vi "message_handle.vi"(0 "Host_Reference":refnum<class "HGF_Reference.lvclass">, 2 "MoAgSy_Message":refnum<class "MoAgSy_Message.lvclass">, 5 "error in (no error)":errorcluster, 8 "timeout in ms (-1)":i32=100) -> (14 "dup Host_Reference":refnum<class "HGF_Reference.lvclass">, 19 "error out":errorcluster)   [LabVIEW 2009, in "MoAgSy.lvlib" / "MoAgSy_Host.lvclass"]
doc: "<B>public</B> VI handels incoming host messages.\n<B>still in progress\nHandles only travel request messages yet</B>\n\nF.Berck@gsi.de\nGSI Darmstadt 2009"
uses:
  MoAgSy_Host.lvclass
  HGF_BaseClasses/HGF_Reference/HGF_Reference.lvclass
  MoAgSy_Message/MoAgSy_Message.lvclass
  HGF_BaseClasses/HGF_Factory/HGF_Factory.lvclass
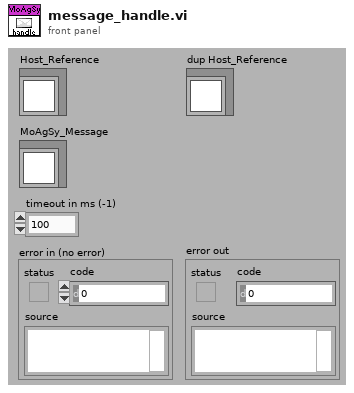
[diagram p1: front panel]
types:
  T1 = enum16{"Not a visitable", "Agent blacklisted", "Host full", "ok"}
  T2 = enum16{"Not a visitable", "Agent blacklisted", "Host full", "ok", "Class Unknown"}
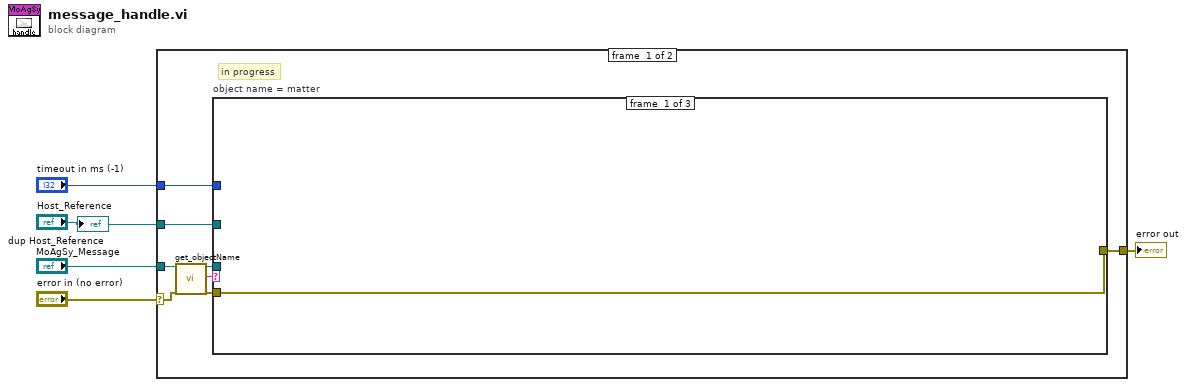
[diagram p0: block diagram]
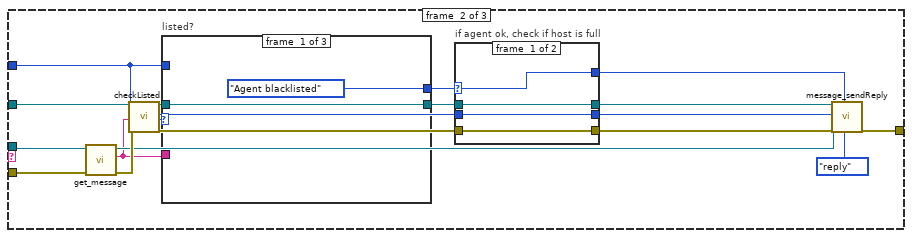
[diagram p2: hidden frame]
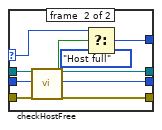
[diagram p3: hidden frame]
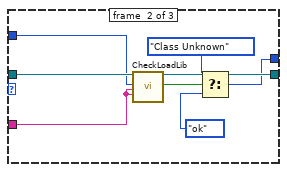
[diagram p4: hidden frame]
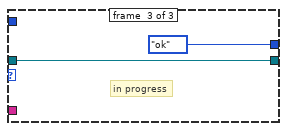
[diagram p5: hidden frame]
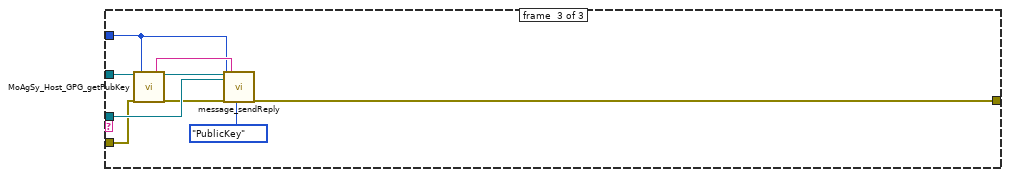
[diagram p6: hidden frame]
diagram:
  n1 = case shown="No Error" "error in (no error)" {
    selector: "error in (no error)" -> [w10 w69]
    tunnel: "MoAgSy_Message" -> [w13 _]
    tunnel: "timeout in ms (-1)" -> [w7 _]
    tunnel: "Host_Reference" -> [w8 _]
    tunnel: [w6 w69] -> w1
    frame #0 {
      # "in progress"
      n2 = call "get_objectName.vi"("HGF_Factory"=w13, "error in (no error)"=w10) -> ("dup HGF_Factory"=w11:refnum<class "MoAgSy_Message.lvclass">, "objectName"=w12:string, "error out"=w9:errorcluster)  [unwired: 15 out]
      n3 = case "object name = matter" shown="\"travel request\"" w12 {
        tunnel: w11 -> [_ w31 w67]
        tunnel: w9 -> [w14 w30 w65]
        tunnel: w8 -> [_ w33 w66]
        tunnel: w7 -> [_ w16 w61]
        tunnel: [w14 w32 w68] -> w6
        frame #0 {
        }
        frame #1 {
          n4 = call "get_message.vi"("error in (no error)"=w30, "MoAgSy_Message.lvclass in"=w31) -> ("error out"=w28:errorcluster, "Message"=w17:string, "MoAgSy_Message.lvclass out"=w27:refnum<class "MoAgSy_Message.lvclass">)  [unwired: 7 out]
          n5 = call "checkListed.vi"("Host_Reference"=w33, "timeout in ms (-1)"=w16, "Library"=w17, "error in (no error)"=w28) -> ("dup Host_Reference"=w18:refnum<class "HGF_Reference.lvclass">, "dup timeout in ms (-1)"=w24:i32, "listed?"=w29:enum16{"blacklisted", "whitelisted", "unlisted"}, "error out"=w22:errorcluster)  [unwired: 12 out]
          n6 = case "listed?" shown="\"whitelisted\"" w29 {
            tunnel: [T1."Agent blacklisted" ("message") w53 T1."ok" ("message")] -> w26
            tunnel: w18 -> [w48 w57 w58]
            tunnel: w17 -> [_ w52 _]
            tunnel: w16 -> [_ w56 _]
            tunnel: [w48 w54 w58] -> w15
            frame #0 {
            }
            frame #1 {
              n7 = call "CheckLoadLib.vi"("Host_Reference"=w57, "timeout in ms (-1)"=w56, "LibraryName"=w52, "classname"=w52) -> ("dup Host_Reference"=w54:refnum<class "HGF_Reference.lvclass">, "status"=w55:bool)  [unwired: 14 in]
              n8 = Select(t=T2."Class Unknown" ("f"), s=w55, f=T1."ok" ("message")) -> (s? t:f=w53:T2)
            }
            frame #2 {
              # "in progress"
            }
          }
          n9 = case "if agent ok, check if host is full" shown="\"Agent blacklisted\", Default" w26 {
            selector: w26 -> [w34 w41]
            tunnel: w15 -> [w37 w47]
            tunnel: [w37 w46] -> w25
            tunnel: w24 -> [w36 w45]
            tunnel: [w36 w44] -> w23
            tunnel: w22 -> [w35 w43]
            tunnel: [w35 w42] -> w21
            tunnel: [w34 w38] -> w20
            frame #0 {
            }
            frame #1 {
              n10 = call "checkHostFree.vi"("Host_Reference"=w47, "timeout in ms (-1)"=w45, "error in (no error)"=w43) -> ("dup Host_Reference"=w46:refnum<class "HGF_Reference.lvclass">, "dup timeout in ms (-1)"=w44:i32, "free4agents"=w39:bool, "error out"=w42:errorcluster)  [unwired: 13 out]
              n11 = Select(t=w41, s=w39, f=T1."Host full") -> (s? t:f=w38:T2)
            }
          }
          n12 = call "message_sendReply.vi"("Host_Reference"=w25, "MoAgSy_Message"=w27, "timeout in ms (-1)"=w23, "error in (no error)"=w21, "message"=w20, "Message Type"=enum16{"error Reply", "reply", "PublicKey"}."reply") -> ("error out"=w32:errorcluster)  [unwired: 1 in, 12 out]
        }
        frame #2 {
          n13 = call "MoAgSy_Host_GPG_getPubKey.vi"("Host_Reference"=w66, "error in (no error)"=w65, "timeout in ms (-1)"=w61) -> ("dup Host_Reference"=w63:refnum<class "HGF_Reference.lvclass">, "public Key"=w64:string, "error out"=w62:errorcluster)  [unwired: 14 in]
          n14 = call "message_sendReply.vi"("Host_Reference"=w63, "MoAgSy_Message"=w67, "timeout in ms (-1)"=w61, "error in (no error)"=w62, "Message"=w64, "Message Type"=enum16{"error Reply", "reply", "PublicKey"}."PublicKey") -> ("error out"=w68:errorcluster)  [unwired: 1 in, 12 out]
        }
      }
    }
    frame #1 {
    }
  }
  "error out" <- w1
  "dup Host_Reference" <- "Host_Reference"
